vi "WilliamPI_CameraSend Images To PC Loop.vi"(8 "error in (no error)":errorcluster, 11 "CameraDevRef":T1) -> ()   [LabVIEW 2015]
doc: "This VI is used to send images to the dashboard using the second enet port on the 8 slot controller. This is provided for compatibility, but is higher overhead than using the Camera MJPG approach.\n\nThis software is licensed. Open the labview\\readme\\WPI Robotics Library Open Source License.txt file for more information."
uses:
  <vilib>/Rock Robotics/WPI/Camera/WPI_CameraImageSize.ctl
  <vilib>/Rock Robotics/WPI/Camera/WPI_CameraDevRef.ctl
  <vilib>/Rock Robotics/WPI/Camera/WPI_CameraWhite Balance Values.ctl
  <vilib>/Rock Robotics/WPI/Camera/WPI_CameraExposure Values.ctl
  <vilib>/Rock Robotics/WPI/Camera/WPI_CameraFrameRate.ctl
  <vilib>/Rock Robotics/SystemInterfaces/NetworkCommunication/NetComm_UsageReport_ResourceType.ctl
  Robot Global Data.vi
panel:
  in  "Image Size 2":T2=enum."320x240"
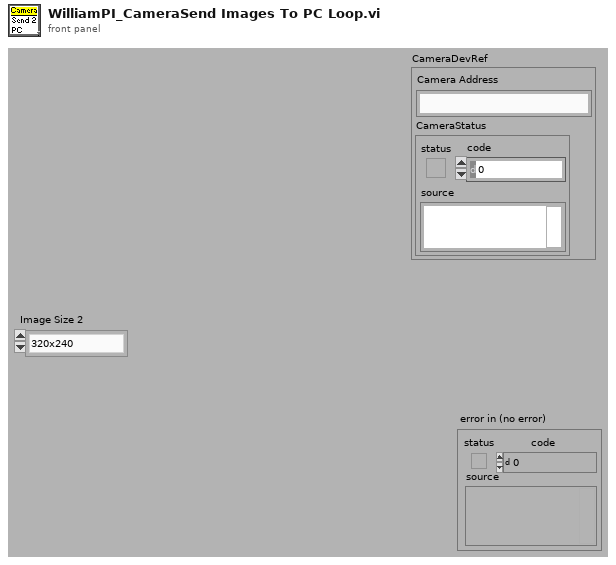
[diagram p1: front panel]
types:
  T1 = typedef "WPI_CameraDevRef.ctl" = cluster{"Camera Address":string, "CameraStatus":errorcluster}
  T2 = typedef "WPI_CameraImageSize.ctl" = enum16{"640x480", "320x240", "160x120", "Custom"}
  T3 = typedef "WPI_CameraFrameRate.ctl" = u32
  T4 = typedef "WPI_CameraExposure Values.ctl" = enum16{"Auto", "Flicker-free 50 Hz", "Flicker-free 60 Hz", "Hold current", "Custom"}
  T5 = typedef "WPI_CameraWhite Balance Values.ctl" = enum16{"Auto", "Fixed indoor", "Fixed outdoor 1", "Fixed outdoor 2", "Fixed fluorescent 1", "Fixed fluorescent 2", "Hold current", "Custom"}
  T6 = cluster{"fps":i32, "compression":i32, "compression 2":i32}
  T7 = typedef "NetComm_UsageReport_ResourceType.ctl" = enum8{"Controller", "Module", "Language", "CANPlugin", "Accelerometer", "ADXL345", "AnalogChannel", "AnalogTrigger", "AnalogTriggerOutput", "CANJaguar", "Compressor", "Counter", "Dashboard", "DigitalInput", "DigitalOutput", "DriverStationCIO", "DriverStationEIO", "DriverStationLCD", "Encoder", "GearTooth", "Gyro", "I2C", "Framework", "Jaguar", "Joystick", "Kinect", "KinectStick", "PIDController", "Preferences", "PWM", "Relay", "RobotDrive", "SerialPort", "Servo", "Solenoid", "SPI", "Task", "Ultrasonic", "Victor", "Button", "Command", "AxisCamera", "PCVideoServer", "SmartDashboard", "Talon", "HiTechnicColorSensor", "HiTechnicAccel", "HiTechnicCompass", "SRF08", "AnalogOutput", "Victor SP", "Talon SRX", "CAN Talon SRX", "ADXL362 Accel", "ADXRS450 Gyro", "Rev SPARK", "Mindsensors SD540", "Digital Filter"}
  T8 = enum16{"Update Mode", "Get Image", "Get Image Data"}
  T9 = typedef "Image Type" = u32
  T10 = typedef "IMAQ Image.ctl" = refnum<image>
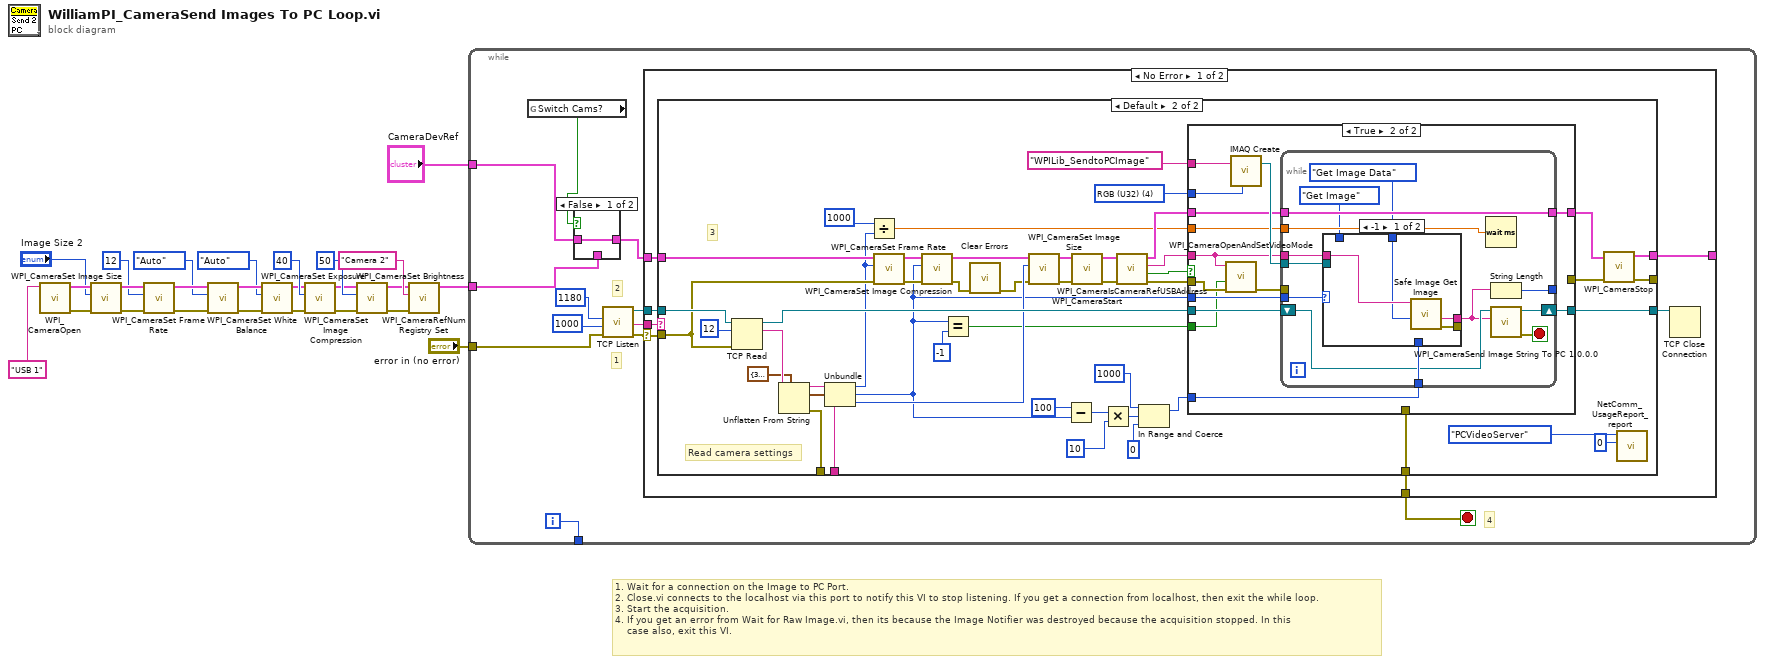
[diagram p0: block diagram]
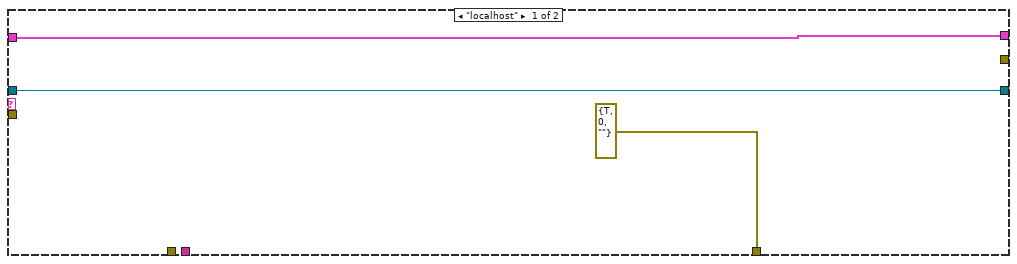
[diagram p3: hidden frame]
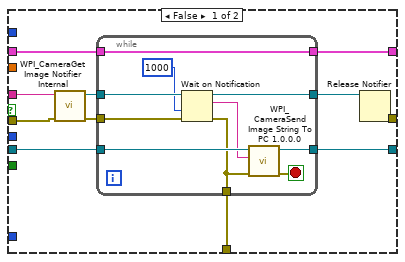
[diagram p4: hidden frame]
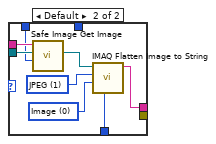
[diagram p5: hidden frame]
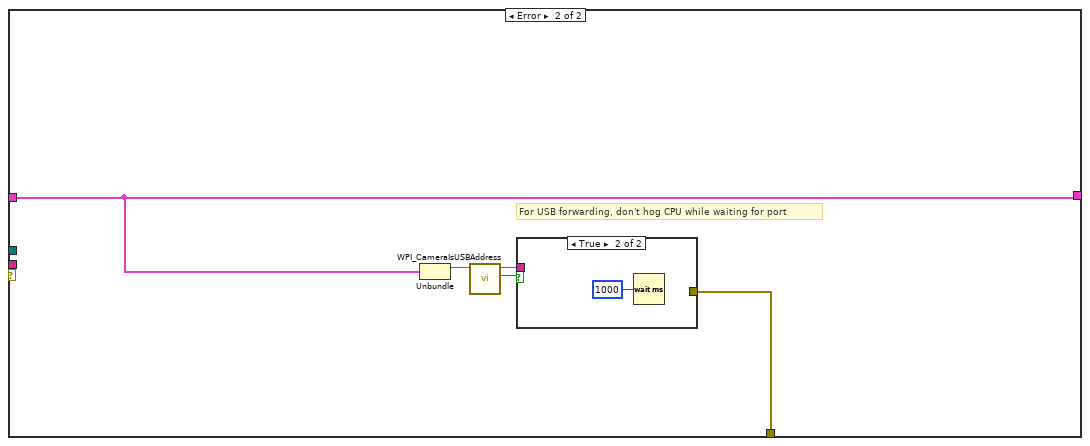
[diagram p6: hidden frame]
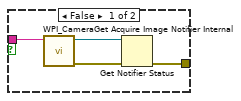
[diagram p7: hidden frame]
diagram:
  # "1. Wait for a connection on the Image to PC Port.\n2. Close.vi connects to the localhost via this port to notify this VI to stop listening. If you get a connection from localhost, then exit the while loop.\n3. Start the acquisition.\n4. If you get an error from Wait for Raw Image.vi, then its because the Image Notifier was destroyed because the acquisition stopped. In this\n    case also, exit this VI."
  n1 = call <vilib>:"WPI_CameraOpen.vi"("Camera Address"="USB 1") -> ("error out"=w15:errorcluster, "CameraDevRef"=w16:T1)  [unwired: 1 in, 8 out]
  n2 = call <vilib>:"WPI_CameraSet Image Size.vi"("error in (no error)"=w15, "Image Size"="Image Size 2", "CameraDevRef"=w16) -> ("error out"=w14:errorcluster, "CameraDevRef Out"=w17:T1)  [unwired: 1 in, 6 out]
  n3 = call <vilib>:"WPI_CameraSet Frame Rate.vi"("error in (no error)"=w14, "Frame Rate (fps)"=T3 12, "CameraDevRef"=w17) -> ("error out"=w13:errorcluster, "CameraDevRef Out"=w19:T1)  [unwired: 7 out]
  n4 = call <vilib>:"WPI_CameraSet White Balance.vi"("error in (no error)"=w13, "White Balance"=WPI_CameraWhite_Balance_Values."Auto", "CameraDevRef"=w19) -> ("error out"=w12:errorcluster, "CameraDevRef Out"=w18:T1)  [unwired: 1 in, 6 out]
  n5 = call <vilib>:"WPI_CameraSet Exposure.vi"("error in (no error)"=w12, "Exposure"=WPI_CameraExposure_Values."Auto", "CameraDevRef"=w18) -> ("error out"=w11:errorcluster, "CameraDevRef Out"=w21:T1)  [unwired: 1 in, 6 out]
  n6 = call <vilib>:"WPI_CameraSet Image Compression.vi"("error in (no error)"=w11, "Compression"=40, "CameraDevRef"=w21) -> ("error out"=w10:errorcluster, "CameraDevRef Out"=w20:T1)  [unwired: 7 out]
  n7 = call <vilib>:"WPI_CameraSet Brightness.vi"("error in (no error)"=w10, "Brightness"=50, "CameraDevRef"=w20) -> ("error out"=w8:errorcluster, "CameraDevRef Out"=w9:T1)  [unwired: 7 out]
  n8 = call <vilib>:"WPI_CameraRefNum Registry Set.vi"("error in (no error)"=w8, "refnum name"="Camera 2", "CameraDevRef"=w9) -> ("CameraDevRef"=w3:T1)  [unwired: 1 in, 7 out]
  n9 = while {
    tunnel: "error in (no error)" -> [w36]
    tunnel: [w30] -> _
    tunnel: w3 -> [w28]
    tunnel: "CameraDevRef" -> [w27]
    i -> [w30]
    stop <- w34 stop-if-true
    # "4"
    # "1"
    # "2"
    n10 = global read "Robot Global Data.vi" "Switch Cams?"() -> (w26:bool)
    n11 = case shown="False" w26 {
      tunnel: [w38 w39] -> w29
      tunnel: w28 -> [_ w39]
      tunnel: w27 -> [w38 _]
      frame False {
      }
      frame True {
      }
    }
    n12 = call <vilib>:"TCP Listen.vi"("error in (no error)"=w36, "timeout ms (wait forever: -1)"=u16 1000 ("port"), "port"=u16 1180) -> ("error out"=w32:errorcluster, "remote address"=w37:string, "connection ID"=w35:refnum<k5>)  [unwired: 1 in, 5 out]
    n13 = case shown="No Error" w32 {
      selector: w32 -> [w40 _]
      tunnel: [w46 w160] -> _
      tunnel: w37 -> [w45 _]
      tunnel: w29 -> [w44 w160]
      tunnel: w35 -> [w43 _]
      tunnel: [w42 w161] -> w34
      frame No Error {
        n14 = case shown="Default" w45 {
          tunnel: [w49 w94] -> w46
          tunnel: w44 -> [w49 w76]
          tunnel: w40 -> [_ w72]
          tunnel: w43 -> [w47 w80]
          tunnel: [errorcluster {"status"=TRUE, "code"=0, "source"=""} ("error out 2") w96] -> w42
          tunnel: [w47 w95] -> w41
          tunnel: [_ w93] -> _
          tunnel: [_ w51] -> _
          tunnel: [_ w50] -> _
          frame "localhost" {
          }
          frame Default {
            w87 = T9 4 items=["Grayscale (U8)", "Grayscale (I16)", "Grayscale (SGL)", "Complex (CSG)", "RGB (U32)", "HSL (U32)", "RGB (U64)", "Grayscale (U16)"] ("Image Type")
            # "Read camera settings"
            # "3"
            n15 = TCP Read(connection ID=w80, bytes to read=12, error in (no error)=w72) -> (connection ID out=w79:refnum<k5>, data out=w77:string)  [unwired: 2 in, 1 out]
            n16 = Unflatten From String(type=T6 {"fps"=30, "compression"=32, "compression 2"=32} ("Camera Settings"), binary string=w77) -> (rest of the binary string=w50:string, value=w69:T6, error out=w51:errorcluster)  [unwired: 3 in]
            n17 = Unbundle(w69) -> ("fps"=w66:i32, "compression"=w55:i32, "compression 2"=w68:i32)
            n18 = Divide(x=u16 1000 ("port"), y=w66) -> (x/y=w65:dbl)
            n19 = call <vilib>:"WPI_CameraSet Frame Rate.vi"("error in (no error)"=w72, "Frame Rate (fps)"=w66, "CameraDevRef"=w76) -> ("error out"=w71:errorcluster, "CameraDevRef Out"=w75:T1)  [unwired: 7 in]
            n20 = call <vilib>:"WPI_CameraSet Image Compression.vi"("error in (no error)"=w71, "Compression"=w55, "CameraDevRef"=w75) -> ("error out"=w53:errorcluster, "CameraDevRef Out"=w74:T1)  [unwired: 7 in]
            n21 = Equal?(x=w55, y=-1) -> (x = y?=w54:bool)
            n22 = call <vilib>:"Clear Errors.vi"("error in (no error)"=w53) -> ("error out"=w52:errorcluster)  [unwired: 5 in, 1 out]
            n23 = call <vilib>:"WPI_CameraSet Image Size.vi"("error in (no error)"=w52, "Image Size"=w68, "CameraDevRef"=w74) -> ("error out"=w70:errorcluster, "CameraDevRef Out"=w73:T1)  [unwired: 7 in]
            n24 = Subtract(x=100, y=w55) -> (x-y=w60:i32)
            n25 = call <vilib>:"WPI_CameraStart.vi"("error in (no error)"=w70, "CameraDevRef"=w73) -> ("error out"=w84:errorcluster, "CameraDevRef"=w82:T1)  [unwired: 8 out]
            n26 = Multiply(x=w60, y=10) -> (x*y=w62:i32)
            n27 = call <vilib>:"WPI_CameraIsCameraRefUSBAddress.vi"("error in (no error)"=w84, "CameraDevRef"=w82) -> ("error out"=w83:errorcluster, "USB?"=w85:bool, "Camera Address Out"=w86:string, "CameraDevRef out"=w81:T1)  [unwired: 6 in]
            n28 = In Range and Coerce(upper limit=1000, x=w62, lower limit=0) -> (coerced(x)=w58:i32)  [unwired: 1 out]
            n29 = case shown="True" w85 {
              tunnel: w79 -> [w107 w131]
              tunnel: [w106 _] -> w96
              tunnel: [w105 w130] -> w95
              tunnel: w83 -> [w104 w121]
              tunnel: w86 -> [w102 w120]
              tunnel: [w101 w125] -> w92
              tunnel: w81 -> [w100 w126]
              tunnel: [w98 _] -> w91
              tunnel: "WPILib_SendtoPCImage" -> [_ w128]
              tunnel: w87 -> [_ w127]
              tunnel: w58 -> [_ w124]
              tunnel: w65 -> [_ w123]
              tunnel: w55 -> [_ w122]
              tunnel: w54 -> [_ w118]
              frame False {
                n30 = call <vilib>:"WPI_CameraGet Image Notifier Internal.vi"("error in (no error)"=w104, "Camera Address"=w102) -> ("error out"=w103:errorcluster, "Image Notifier"=w99:refnum<notifier>)  [unwired: 8 out]
                n31 = while {
                  tunnel: w103 -> [w113]
                  tunnel: w107 -> [w117]
                  tunnel: [w110] -> w106
                  tunnel: [w115] -> w105
                  tunnel: [w114] -> w101
                  tunnel: w100 -> [w114]
                  tunnel: w99 -> [w112]
                  tunnel: [w108] -> w97
                  stop <- w116 stop-if-true
                  n32 = Wait on Notification(notifier=w112, timeout in ms (-1)=1000 ("Timeout in ms (-1)"), error in (no error)=w113) -> (notifier out=w108:refnum<notifier>, notification=w111:string, error out=w110:errorcluster)  [unwired: 2 out]
                  n33 = call <vilib>:"WPI_CameraSend Image String To PC 1.0.0.0.vi"("error in (no error)"=w110, "String"=w111, "TCP Connection ID"=w117) -> ("error out"=w116:errorcluster, "TCP Connection ID out"=w115:refnum<k5>)  [unwired: 7 out]
                }
                n34 = Release Notifier(notifier=w97) -> (error out=w98:errorcluster)  [unwired: 1 in, 3 out]
              }
              frame True {
                n35 = call <vilib>:"WPI_CameraOpenAndSetVideoMode.vi"("error in (no error)"=w121, "USB JPEG"=w118, "Camera Address Out"=w120) -> ("error out"=w119:errorcluster)  [unwired: 8 in]
                n36 = call "IMAQ Create"("Image Name"=w128, "Image Type"=w127) -> ("New Image"=w129:T10)  [unwired: 3 in, 1 out]
                n37 = while {
                  tunnel: w120 -> [w143]
                  shift-right: [w144] -> w130
                  shift-left: w131 -> [w137]
                  tunnel: w129 -> [w142]
                  tunnel: [w140] -> w125
                  tunnel: w126 -> [w140]
                  tunnel: w124 -> [w139]
                  tunnel: w123 -> [w138]
                  tunnel: [w135] -> _
                  tunnel: w122 -> [w134]
                  tunnel: w119 -> [_]
                  stop <- w141 stop-if-true
                  n38 = case shown="-1" w134 {
                    tunnel: [w147 w156] -> w136
                    tunnel: w143 -> [w148 w152]
                    tunnel: w142 -> [_ w151]
                    tunnel: w139 -> [_ w153]
                    tunnel: [w146 _] -> _
                    tunnel: T8."Get Image Data" ("Operation") -> [w145 _]
                    tunnel: T8."Get Image" ("Operation") -> [_ w149]
                    frame -1 {
                      n39 = call <vilib>:"Safe Image Get Image.vi"("Operation"=w145, "Session In"=w148) -> ("error out"=w146:errorcluster, "Image Data String"=w147:string)  [unwired: 6 in, 2 out]
                    }
                    frame Default {
                      w154 = 0 items=["Image", "Image and Vision Info", "Reference to Image"] ("Type of Flatten (Image and Vision Info)")
                      w155 = 1 items=["None", "JPEG", "PACKED BINARY"] ("Compression (None)")
                      n40 = call <vilib>:"Safe Image Get Image.vi"("Operation"=w149, "Image In"=w151, "Session In"=w152) -> ("Image Out"=w150:T10)  [unwired: 5 in, 3 out]
                      n41 = call "IMAQ Flatten Image to String"("Quality (750)"=w153, "Type of Flatten (Image and Vision Info)"=w154, "Compression (None)"=w155, "Image"=w150) -> ("Data String"=w156:string)  [unwired: 6 in, 1 out]
                    }
                  }
                  n42 = Wait (ms)(milliseconds to wait=w138) -> ()  [unwired: 1 out]
                  n43 = String Length(string=w136) -> (length=w135:i32)
                  n44 = call <vilib>:"WPI_CameraSend Image String To PC 1.0.0.0.vi"("String"=w136, "TCP Connection ID"=w137) -> ("error out"=w141:errorcluster, "TCP Connection ID out"=w144:refnum<k5>)  [unwired: 1 in, 7 out]
                }
              }
            }
            n45 = call <vilib>:"WPI_CameraStop.vi"("error in (no error)"=w91, "CameraDevRef"=w92) -> ("error out"=w93:errorcluster, "CameraDevRef"=w94:T1)  [unwired: 8 out]
            n46 = call <vilib>:"NetComm_UsageReport_report.vi"("Instance Number"=u8 0, "Resource Type"=NetComm_UsageReport_ResourceType."PCVideoServer") -> ()  [unwired: 10 in]
          }
        }
        n47 = TCP Close Connection(connection ID=w41) -> ()  [unwired: 1 in, 3 out]
      }
      frame Error {
        # "For USB forwarding, don't hog CPU while waiting for port"
        n48 = Unbundle(w160) -> ("Camera Address"=w159:string)  [unwired: 1 out]
        n49 = call <vilib>:"WPI_CameraIsUSBAddress.vi"("Camera Address In"=w159) -> ("USB?"=w157:bool, "Camera Address Out"=w158:string)  [unwired: 8 in, 1 out]
        n50 = case shown="True" w157 {
          tunnel: [w165 _] -> w161
          tunnel: w158 -> [w162 _]
          frame False {
            n51 = call <vilib>:"WPI_CameraGet Acquire Image Notifier Internal.vi"("Camera Address"=w162) -> ("error out"=w163:errorcluster, "Acquire Image Notifier"=w164:refnum<notifier>)  [unwired: 1 in, 8 out]
            n52 = Get Notifier Status(notifier=w164, error in (no error)=w163) -> (error out=w165:errorcluster)  [unwired: 4 out]
          }
          frame True {
            n53 = Wait (ms)(milliseconds to wait=u32 1000) -> ()  [unwired: 1 out]
          }
        }
      }
    }
  }
